vi "全局 环境参数.vi"() -> ()   [LabVIEW 2016, in "数据传输系统.lvlib"]
panel:
  in  "湿度":string[][](array[string])
  in  "室温":string[][](array[string])
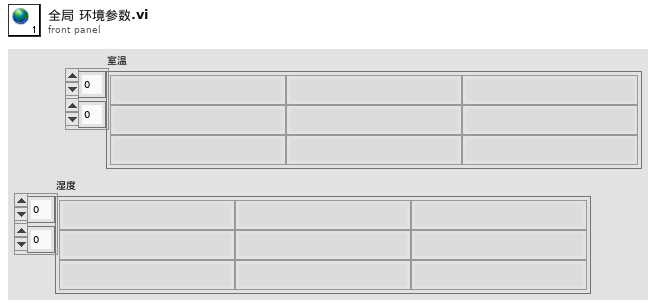
[diagram p1: front panel]
diagram:
